vi "Create Accessors.vi"(10 "LVClassLibrary":refnum<vi>, 11 "Accessor Options":T1) -> ()   [LabVIEW 2018, in "LVClassByRef.lvlib"]
uses:
  <resource>/Framework/Providers/LVClassByRef/LVClassByRef.lvlib
  <resource>/Framework/Providers/LVClassByRef/Accessor Options.ctl
  <resource>/Framework/Providers/LVClassByRef/Setter Template.vit
  <resource>/Framework/Providers/LVClassByRef/Getter Template.vit
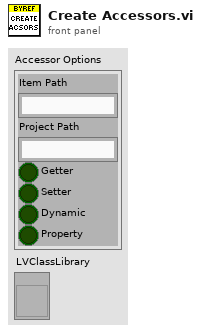
[diagram p1: front panel]
types:
  T1 = typedef "LVClassByRef.lvlib/Accessor Options.ctl" = cluster{"Item Path":string, "Project Path":string, "Getter":bool, "Setter":bool, "Dynamic":bool, "Property":bool}
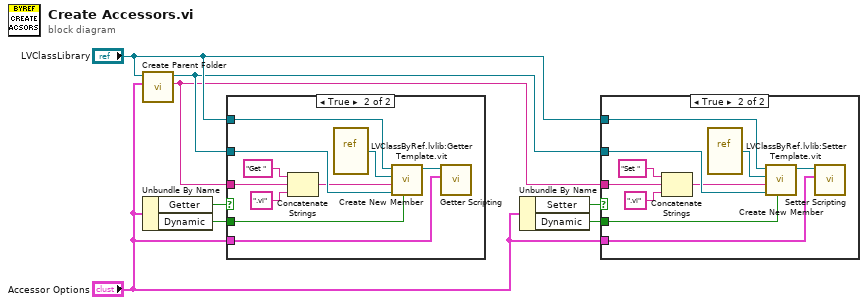
[diagram p0: block diagram]
diagram:
  n1 = call <resource>:"Create Parent Folder.vi"("Accessor Options"="Accessor Options", "LVClassLibrary"="LVClassLibrary") -> ("Item Name"=w4:string, "Parent"=w5:refnum<vi>)  [unwired: 8 in]
  n2 = Unbundle By Name("Accessor Options") -> ("Getter"=w8:bool, "Dynamic"=w7:bool)
  n3 = case shown="True" w8 {
    tunnel: w5 -> [_ w16]
    tunnel: "Accessor Options" -> [_ w14]
    tunnel: "LVClassLibrary" -> [_ w17]
    tunnel: w4 -> [_ w12]
    tunnel: w7 -> [_ w13]
    frame False {
    }
    frame True {
      n4 = Concatenate Strings("Get " ("string"), w12, ".vi" ("string")) -> (w9:string)
      n5 = vi-ref "LVClassByRef.lvlib:Getter Template.vit"() -> (w18:refnum<vi>)
      n6 = call <resource>:"Create New Member.vi"("Dynamic?"=w13, "Parent"=w16, "Name"=w9, "Template"=w18, "LVClassLibrary"=w17) -> ("Member VI"=w15:refnum<vi>)  [unwired: 5 in, 1 out]
      n7 = call <resource>:"Getter Scripting.vi"("Accessor Options"=w14, "VI Refnum"=w15) -> ()  [unwired: 10 in]
    }
  }
  n8 = Unbundle By Name("Accessor Options") -> ("Setter"=w2:bool, "Dynamic"=w1:bool)
  n9 = case shown="True" w2 {
    tunnel: w5 -> [_ w26]
    tunnel: "Accessor Options" -> [_ w24]
    tunnel: "LVClassLibrary" -> [_ w27]
    tunnel: w4 -> [_ w23]
    tunnel: w1 -> [_ w19]
    frame False {
    }
    frame True {
      n10 = Concatenate Strings("Set " ("string"), w23, ".vi" ("string")) -> (w20:string)
      n11 = vi-ref "LVClassByRef.lvlib:Setter Template.vit"() -> (w28:refnum<vi>)
      n12 = call <resource>:"Create New Member.vi"("Dynamic?"=w19, "Parent"=w26, "Name"=w20, "Template"=w28, "LVClassLibrary"=w27) -> ("Member VI"=w25:refnum<vi>)  [unwired: 5 in, 1 out]
      n13 = call <resource>:"Setter Scripting.vi"("Accessor Options"=w24, "VI Refnum"=w25) -> ()  [unwired: 10 in]
    }
  }
